vi "Get Mac Address.vi"(8 "error in (no error)":errorcluster, 11 "buffer":string) -> (0 "error out":errorcluster, 3 "buffer out":string)   [LabVIEW 2015, in "QCA_DUT_Func.lvlib"]
doc: "DLL_QMSL_AEROFLEX void _stdcall GetMacAddress(char *buffer);"
uses:
  QCA_DUT_Func.lvlib
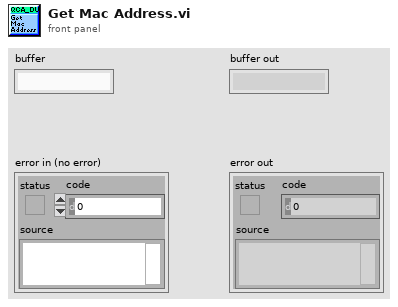
[diagram p1: front panel]
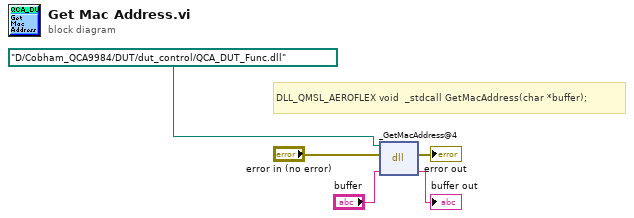
[diagram p0: block diagram]
diagram:
  # "DLL_QMSL_AEROFLEX void  _stdcall GetMacAddress(char *buffer);"
  n1 = dll-call lib="D:/Cobham_QCA9984/VI/QCA_DUT_Func.dll" fn="_GetMacAddress@4"(path in=path "D:/Cobham_QCA9984/DUT/dut_control/QCA_DUT_Func.dll", error in="error in (no error)", "buffer"="buffer") -> (error out=→"error out":errorcluster, "buffer"=→"buffer out":string)  [unwired: 2 in, 1 out]
